vi "RIGOL DG4000 Series Arbitrary Waveform.vi"() -> ()   [LabVIEW 2012]
doc: "This example shows how to create then configure an arbitrary waveform."
uses:
  Instance           2 46Saved   RIGOL DG4000 Series Arbitrary Waveform .vi
  Instance           1 46Saved   RIGOL DG4000 Series Arbitrary Waveform .vi
  <instrlib>/RIGOL DG4000 Series/Public/Configure/Configure Arbitrary Waveform.vi
  <instrlib>/RIGOL DG4000 Series/RIGOL DG4000 Series.lvlib
panel:
  in  "Output Channel (1: Channel 1)":i32(ring)=1 items=["Channel 1"=1, "Channel 2"=2]
  in  "Offset (0.00 V)":dbl
  in  "Frequency (1000 Hz)":dbl=1000.0
  in  "Gain (5.0)":dbl=5.0
  in  "VISA resource name":refnum<visa-resource-name>
  # "(c) 2012 National Instruments.  ALL RIGHTS RESERVED."
  # "To edit the Arbitrary Waveform, use the Simulate Arbitrary Signal on the block diagram."
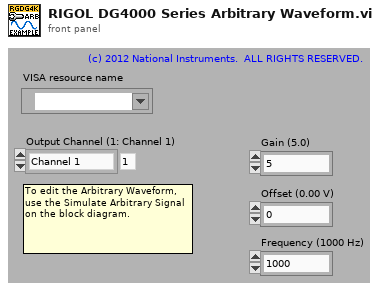
[diagram p1: front panel]
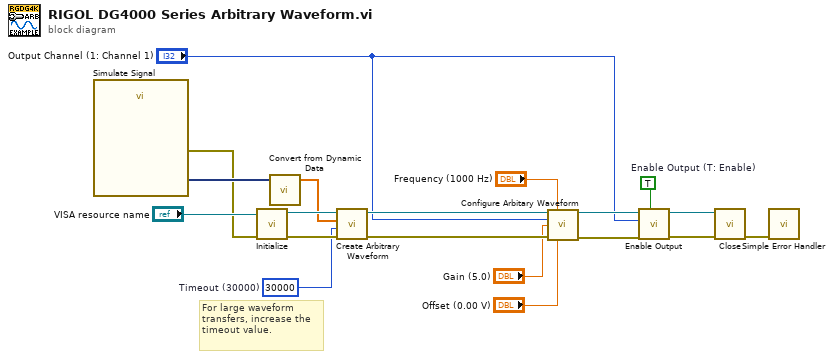
[diagram p0: block diagram]
diagram:
  w3 = TRUE  # Enable Output (T: Enable)
  w1 = u32 30000  # Timeout (30000)
  # "For large waveform transfers, increase the timeout value."
  n1 = call "Simulate Signal"() -> ("Sine with Uniform Noise"=w19:dynamicdata, "error out"=w17:errorcluster)  [unwired: 8 in, 6 out]
  n2 = call <instrlib>:"Initialize.vi"("error in (no error)"=w17, "VISA resource name"="VISA resource name") -> ("error out"=w13:errorcluster, "VISA resource name out"=w12:refnum<visa-resource-name>)  [unwired: 2 in, 6 out]
  n3 = call "Convert from Dynamic Data"("Dynamic Data Type"=w19) -> ("Array"=w4:dbl[])  [unwired: 3 out]
  n4 = call <instrlib>:"Create Arbitrary Waveform.vi"("error in (no error)"=w13, "Timeout (10000 ms)"=w1, "Arbitrary Waveform Data (0)"=w4, "VISA resource name"=w12) -> ("error out"=w8:errorcluster, "VISA resource name out"=w11:refnum<visa-resource-name>)  [unwired: 2 in, 4 out]
  n5 = call "Configure Arbitary Waveform.vi"("VISA resource name"=w11, "Frequency (1000 Hz)"="Frequency (1000 Hz)", "Output Channel (1: Channel 1)"="Output Channel (1: Channel 1)", "Amplitude (5 Vpp)"="Gain (5.0)", "error in (no error)"=w8, "Offset (0)"="Offset (0.00 V)") -> ("VISA resource name out"=w10:refnum<visa-resource-name>, "error out"=w9:errorcluster)  [unwired: 8 in]
  n6 = call <instrlib>:"Enable Output.vi"("Enable Output (T: Enable)"=w3, "error in (no error)"=w9, "Output Channel (1: Channel 1)"="Output Channel (1: Channel 1)", "VISA resource name"=w10) -> ("error out"=w15:errorcluster, "VISA resource name out"=w14:refnum<visa-resource-name>)  [unwired: 6 out]
  n7 = call <instrlib>:"Close.vi"("error in (no error)"=w15, "VISA resource name"=w14) -> ("error out"=w16:errorcluster)  [unwired: 9 out]
  n8 = call <vilib>:"Simple Error Handler.vi"("error in (no error)"=w16) -> ()  [unwired: 1 in, 8 out]
